vi "SV to subscribe to.vi"(8 "error in (no error)":errorcluster, 11 "Father of all uServices in":refnum<class "Father of all uServices.lvclass">) -> (0 "error out":errorcluster, 1 "Needs to Deploy":bool, 2 "SV to subscribe to":string[](array[string]), 3 "Father of all uServices out":refnum<class "Father of all uServices.lvclass">)   [LabVIEW 2020, in "TALOS.lvlib" / "Father of all uServices.lvlib" / "Father of all uServices.lvclass"]
uses:
  Father of all uServices.lvclass
  Ancestor/Ancestor/Ancestor.lvclass/Ancestor.ctl
  <vilib>/AdvancedString/Delimited String to 1D String Array.vi
  Support VIs/Generate Error.vi
  FGV/Error Memory/Get Error Description.vi
  Support VIs/Get PC name.vi
  Ancestor/Ancestor/Read ID.vi
  <vilib>/Utility/error.llb/Clear Errors.vi
  FGV/Error Memory/Error Memory Core.vi
  Support VIs/Circus Root Path.vi
  FGV/Error Memory/Error Crt Lvl checker.vi
  FGV/Error Memory/Error Memory Core.vi/40c8088d-b597-4017-91af-faa98e00292e.vi
  FGV/Error Memory/Error Memory Core.vi/d4a3ab98-063c-4e44-b43d-fbdcfe6c2be2.vi
  <vilib>/Utility/LVClass/Get LV Class Name.vi
  Support VIs/Global Memory.vi
  Support VIs/Is in Packed Library.vi
  Support VIs/TALOS Root path.vi
  Support VIs/Read CSV worksheet.vi
  Support VIs/Global Constants.vi
  <vilib>/Utility/error.llb/General Error Handler.vi
  Support VIs/Error Log.vi
  Ancestor/Ancestor/Ancestor.lvclass
  <vilib>/Comparison/Equal/Equal Functor/Equal Functor.lvclass
  TALOS.lvlib
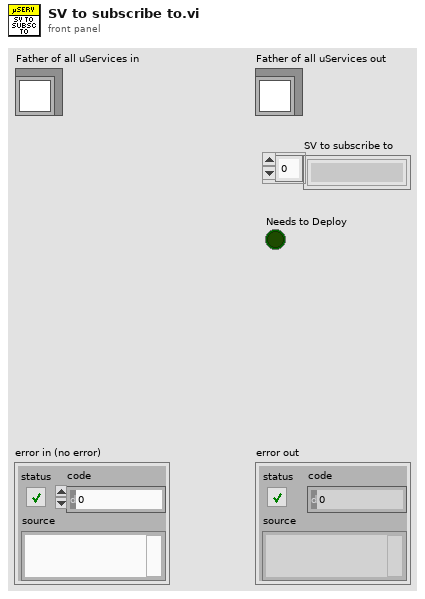
[diagram p1: front panel]
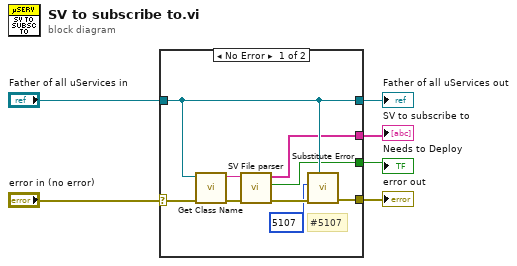
[diagram p0: block diagram]
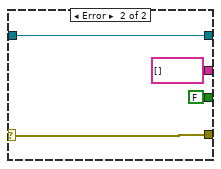
[diagram p2: hidden frame]
diagram:
  n1 = case shown="No Error" "error in (no error)" {
    selector: "error in (no error)" -> [w14 w18]
    tunnel: [w11 string[] [] ("SV to subscribe to")] -> w2
    tunnel: [w9 w18] -> w5
    tunnel: "Father of all uServices in" -> [w15 w19]
    tunnel: [w15 w19] -> w3
    tunnel: [w10 FALSE ("Needs to Deploy")] -> w1
    frame No Error {
      # "#5107"
      n2 = call "Get Class Name.vi"("error in (no error)"=w14, "object"=w15) -> ("error out"=w12:errorcluster, "Class Name"=w13:string)  [unwired: 8 in]
      n3 = call "SV File parser.vi"("error in (no error)"=w12, "uService ID"=w13) -> ("error out"=w8:errorcluster, "Needs to Deploy"=w10:bool, "SV to subscribe to"=w11:string[])  [unwired: 7 in]
      n4 = call "Substitute Error.vi"("LabVIEW Object"=w15, "error in (no error)"=w8, "Error Code"=5107) -> ("error out"=w9:errorcluster)  [unwired: 8 in]
    }
    frame Error {
    }
  }
  "error out" <- w5
  "Father of all uServices out" <- w3
  "SV to subscribe to" <- w2
  "Needs to Deploy" <- w1
